vi "Theme Editor Config--constant.vi"() -> (3 "Button Editor Config":path)   [LabVIEW 2021, in "Theme Config.lvclass"]
doc: "Constant VI to define the location of the theme editor configuration file.\n\n<b>Code Developed By:</b>\nTechnology Service Corporation\nwww.tsc.com/atcs\n\nDeveloper:\nDaniel Coons"
uses:
  Theme Config.lvclass
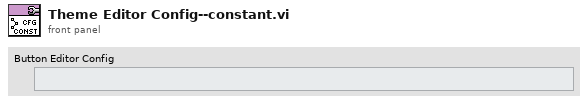
[diagram p1: front panel]
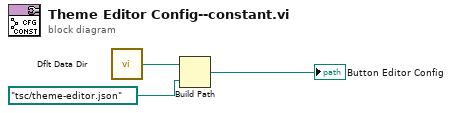
[diagram p0: block diagram]
diagram:
  n1 = call <vilib>:"Dflt Data Dir.vi"() -> ("App:Default Data Directory"=w1:path)
  n2 = Build Path(base path=w1, name or relative path=path "tsc/theme-editor.json") -> (appended path=→"Button Editor Config":path)
